vi "ds18b20.vi"() -> ()   [LabVIEW 2017]
uses:
  <vilib>/Instr/_visa.llb/VISA Configure Serial Port (Instr).vi
panel:
  out "Sıcaklık":u8(slide) scale=0.0..100.0
  out "Low Heat":bool
  out "Ideal Heat":bool
  out "Overheated":bool
  # "BABY FOOD POT"
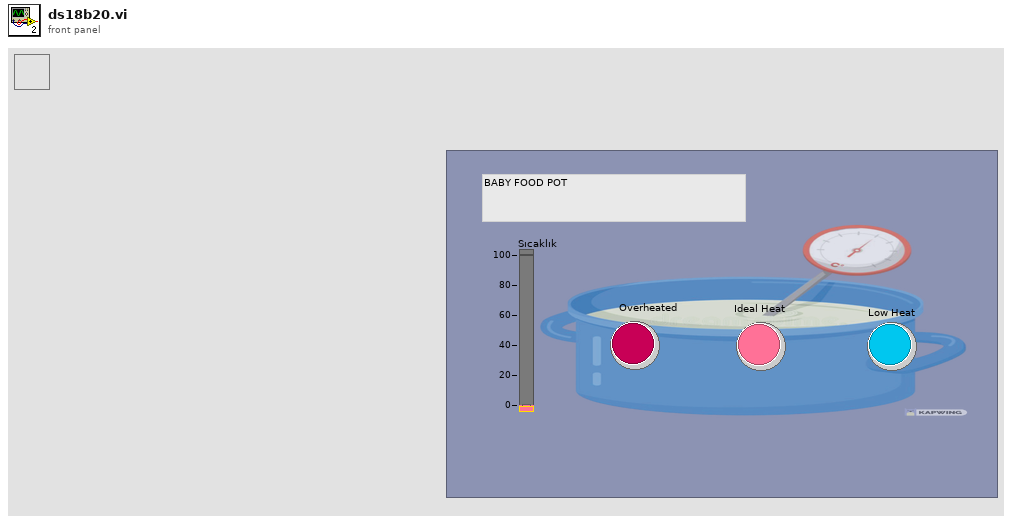
[diagram p1: front panel]
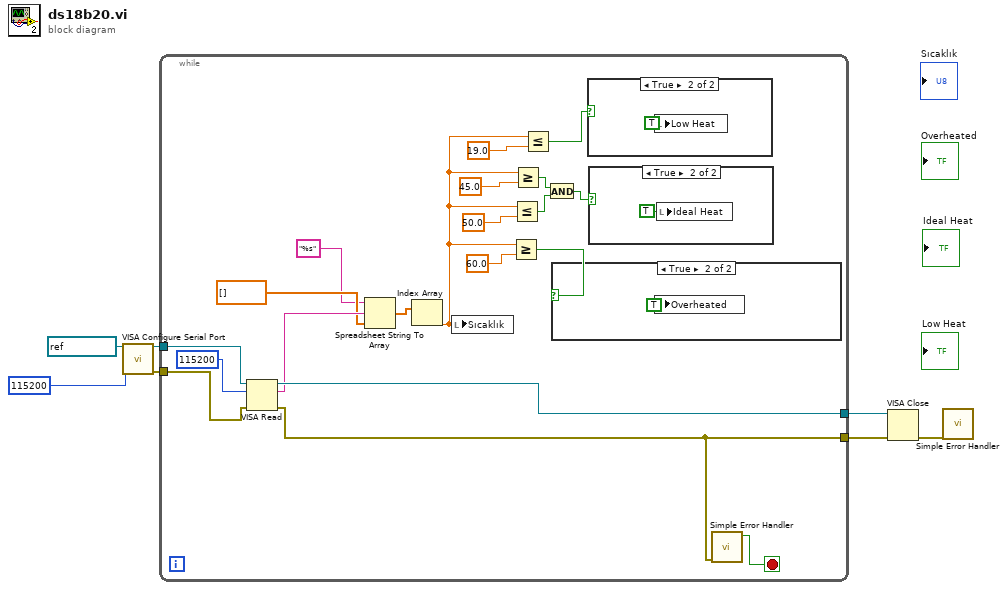
[diagram p0: block diagram]
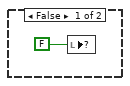
[diagram p2: hidden frame]
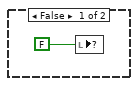
[diagram p3: hidden frame]
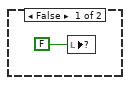
[diagram p4: hidden frame]
diagram:
  n1 = call-poly "VISA Configure Serial Port"("VISA resource name"=refnum<visa-resource-name> "COM5", "baud rate (9600)"=u32 115200) -> ("VISA resource name out"=w5:refnum<visa-resource-name>, "error out"=w7:errorcluster)  [unwired: 12 in]
  n2 = while {
    tunnel: w7 -> [w27]
    tunnel: [w24] -> w6
    tunnel: w5 -> [w26]
    tunnel: [w25] -> w4
    stop <- w23 stop-if-true
    n3 = VISA Read(VISA resource name=w26, byte count=u32 115200 ("baud rate (9600)"), error in (no error)=w27) -> (VISA resource name out=w25:refnum<visa-resource-name>, read buffer=w21:string, error out=w24:errorcluster)  [unwired: 1 out]
    n4 = Spreadsheet String To Array(format string="%s", spreadsheet string=w21, array type (2D Dbl)=dbl[] []) -> (array=w18:dbl[])  [unwired: 1 in]
    n5 = Index Array(array=w18) -> (element=w15:dbl)  [unwired: 1 in]
    n6 = local write "Sıcaklık"(w15) -> ()
    n7 = Greater Or Equal?(x=w15, y=60.0) -> (x >= y?=w8:bool)
    n8 = Less Or Equal?(x=w15, y=50.0) -> (x <= y?=w16:bool)
    n9 = Greater Or Equal?(x=w15, y=45.0) -> (x >= y?=w17:bool)
    n10 = Less Or Equal?(x=w15, y=19.0) -> (x <= y?=w10:bool)
    n11 = And(x=w17, y=w16) -> (x .and. y?=w9:bool)
    n12 = case shown="True" w8 {
      frame False {
        n13 = local write item#-1(FALSE ("Alto")) -> ()
      }
      frame True {
        n14 = local write "Overheated"(TRUE ("Alto")) -> ()
      }
    }
    n15 = case shown="True" w10 {
      frame False {
        n16 = local write item#-1(FALSE ("bajo")) -> ()
      }
      frame True {
        n17 = local write "Low Heat"(TRUE ("bajo")) -> ()
      }
    }
    n18 = case shown="True" w9 {
      frame False {
        n19 = local write item#-1(FALSE ("normal")) -> ()
      }
      frame True {
        n20 = local write "Ideal Heat"(TRUE ("normal")) -> ()
      }
    }
    n21 = call <vilib>:"Simple Error Handler.vi"("error in (no error)"=w24) -> ("error?"=w23:bool)  [unwired: 4 in, 4 out]
  }
  n22 = VISA Close(VISA resource name=w4, error in (no error)=w6) -> (error out=w3:errorcluster)
  n23 = call <vilib>:"Simple Error Handler.vi"("error in (no error)"=w3) -> ()  [unwired: 4 in, 5 out]
